vi "Simulated iRobot Close.vi"(8 "error in":errorcluster, 11 "Cal Climber":T1) -> (0 "error out":errorcluster)   [LabVIEW 2013]
uses:
  Simulated iRobot.ctl
  <instrlib>/DC Motor Controller/HAIOL/DC Motor Controller.lvclass
  <vilib>/robotics/Simulator/NI_Robotics_Simulator.lvlib
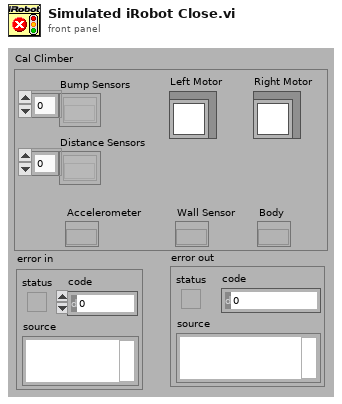
[diagram p1: front panel]
types:
  T1 = typedef "Simulated iRobot.ctl" = cluster{"Bump Sensors":refnum<k20>[], "Distance Sensors":refnum<k20>[], "Accelerometer":refnum<k20>, "Wall Sensor":refnum<k20>, "Body":refnum<k20>, "Left Motor":refnum<class "DC Motor Controller.lvclass">, "Right Motor":refnum<class "DC Motor Controller.lvclass">}
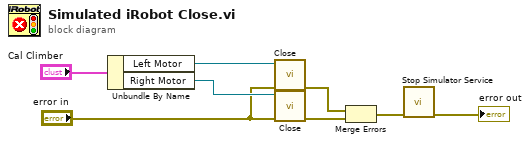
[diagram p0: block diagram]
diagram:
  n1 = Unbundle By Name("Cal Climber") -> ("Left Motor"=w7:refnum<class "DC Motor Controller.lvclass">, "Right Motor"=w6:refnum<class "DC Motor Controller.lvclass">)
  n2 = call-dynamic "Close.vi"("error in (no error)"="error in", "DC Motor Controller in"=w7) -> ("error out"=w4:errorcluster)  [unwired: 9 in]
  n3 = call-dynamic "Close.vi"("error in (no error)"="error in", "DC Motor Controller in"=w6) -> ("error out"=w3:errorcluster)  [unwired: 9 in]
  n4 = Merge Errors(w4, w3) -> (w2:errorcluster)
  n5 = call <vilib>:"Stop Simulator Service.vi"("error in (no error)"=w2) -> ("error out"=→"error out":errorcluster)  [unwired: 10 in]
